vi "Second_VI.vi"() -> ()   [LabVIEW 2011]
panel:
  out "Numeric":dbl
  in  "Knob":dbl(knob) scale=0.0..10.0
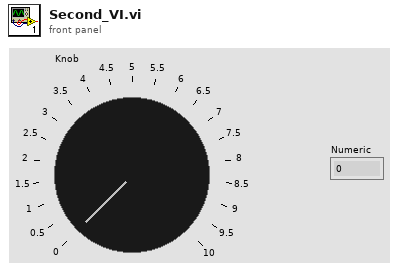
[diagram p1: front panel]
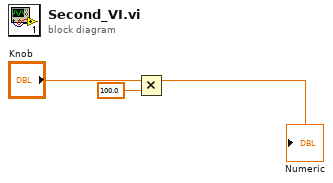
[diagram p0: block diagram]
diagram:
  n1 = Multiply(x="Knob", y=100.0) -> (x*y=→"Numeric":dbl)
